vi "Simple Add.vi"() -> ()   [LabVIEW 2018]
panel:
  out "x+y 2":dbl
  in  "y":dbl
  out "x+y":dbl
  in  "x":dbl
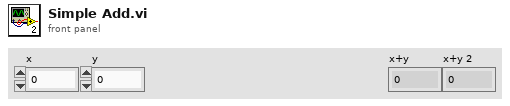
[diagram p1: front panel]
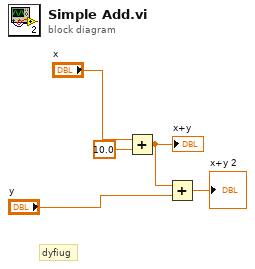
[diagram p0: block diagram]
diagram:
  # "dyfiug"
  n1 = Add(x="x", y=10.0) -> (x+y=w3:dbl)
  "x+y" <- w3
  n2 = Add(x=w3, y="y") -> (x+y=→"x+y 2":dbl)
